vi "Timing_information.vi"(10 "end value (standard value = -31999)":i16=-31999, 11 "starting value (standard value = -2000)":i16=-2000) -> (0 "4bit":i16, 1 "3bit":i16, 2 "2bit":i16, 3 "1bit":i16)   [LabVIEW 2012]
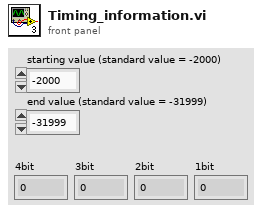
[diagram p1: front panel]
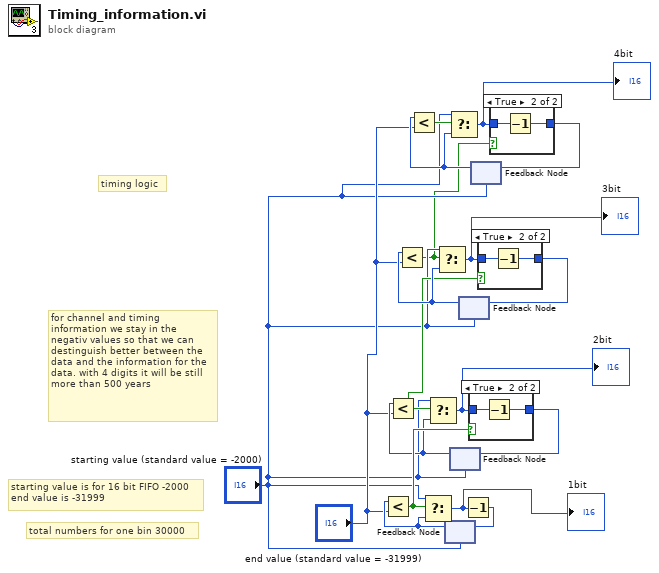
[diagram p0: block diagram]
diagram:
  # "for channel and timing information we stay in the negativ values so that we can destinguish better between the data and the information for the data. with 4 digits it will be still more than 500 years"
  # "total numbers for one bin 30000"
  # "starting value is for 16 bit FIFO -2000\nend value is -31999"
  # "timing logic"
  n1 = feedback #1("starting value (standard value = -2000)") -> (w13:i16)
  n2 = Less?(x=w13, y="end value (standard value = -31999)") -> (x < y?=w14:bool)
  n3 = Select(t="starting value (standard value = -2000)", s=w14, f=w13) -> (s? t:f=w17:i16)
  "1bit" <- w17
  n4 = feedback #2("starting value (standard value = -2000)") -> (w12:i16)
  n5 = Less?(x=w12, y="end value (standard value = -31999)") -> (x < y?=w8:bool)
  n6 = Select(t="starting value (standard value = -2000)", s=w8, f=w12) -> (s? t:f=w16:i16)
  "2bit" <- w16
  n7 = feedback #3("starting value (standard value = -2000)") -> (w11:i16)
  n8 = Less?(x=w11, y="end value (standard value = -31999)") -> (x < y?=w1:bool)
  n9 = Select(t="starting value (standard value = -2000)", s=w1, f=w11) -> (s? t:f=w9:i16)
  "3bit" <- w9
  n10 = Decrement(x=w17) -> (x-1=w18:i16)
  n11 = feedback-in #1(w18) -> ()
  n12 = case shown="True" w14 {
    tunnel: w16 -> [w19 w21]
    tunnel: [w19 w20] -> w15
    frame False {
    }
    frame True {
      n13 = Decrement(x=w21) -> (x-1=w20:i16)
    }
  }
  n14 = feedback-in #2(w15) -> ()
  n15 = feedback #4("starting value (standard value = -2000)") -> (w4:i16)
  n16 = Less?(x=w4, y="end value (standard value = -31999)") -> (x < y?=w7:bool)
  n17 = Select(t="starting value (standard value = -2000)", s=w7, f=w4) -> (s? t:f=w6:i16)
  "4bit" <- w6
  n18 = case shown="True" w8 {
    tunnel: w9 -> [w22 w24]
    tunnel: [w22 w23] -> w10
    frame False {
    }
    frame True {
      n19 = Decrement(x=w24) -> (x-1=w23:i16)
    }
  }
  n20 = feedback-in #3(w10) -> ()
  n21 = case shown="True" w1 {
    tunnel: w6 -> [w25 w27]
    tunnel: [w25 w26] -> w5
    frame False {
    }
    frame True {
      n22 = Decrement(x=w27) -> (x-1=w26:i16)
    }
  }
  n23 = feedback-in #4(w5) -> ()
